vi "GCSArray_regex_string.vi"(0 "Selector":T1, 5 "error in (no error)":errorcluster) -> (14 "Regex string":string, 19 "error out":errorcluster)   [LabVIEW 2026]
doc: "Translates a GCSArray_regex_selector value into its corresponding regular expression string (regex). These text string expressions are used to filter, cut and select text areas in GCS arrays with the LabVIEW regular expression engine.\n\nFor details on how it works, please visit:\nhttps://zone.ni.com/reference/en-XX/help/371361L-01/glang/match_regular_expression/"
uses:
  GCSArray_regex_selector.ctl
panel:
  # "Translate a GCSArray selector enum value into the\ncorresponding regular expression string."
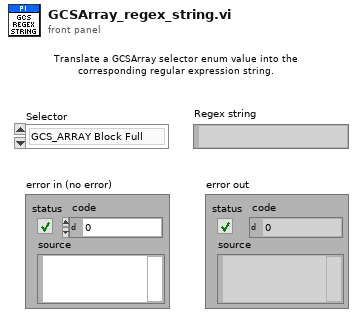
[diagram p1: front panel]
types:
  T1 = typedef "GCSArray_regex_selector.ctl" = enum16{"GCS_ARRAY Block Full", "GCS_ARRAY Block ID", "GCS_ARRAY Block Header", "GCS_ARRAY Block Data", "GCS_ARRAY Identifier", "GCS_ARRAY Remark", "GCS_ARRAY Version", "GCS_ARRAY Dimension", "GCS_ARRAY Type", "GCS_ARRAY Separator", "GCS_ARRAY NData", "GCS_ARRAY NData%", "GCS_ARRAY NData% Keyword", "GCS_ARRAY Name%", "GCS_ARRAY Name% Keyword", "GCS_ARRAY Start%", "GCS_ARRAY Start% Keyword", "GCS_ARRAY End%", "GCS_ARRAY End% Keyword", "GCS_ARRAY Delta%", "GCS_ARRAY Delta% Keword", "GCS_ARRAY Sample Time", "GCS_ARRAY Unit of transmitted value%", "GCS_ARRAY Trans_Unit% Keyword", "GCS_ARRAY Trans_Unit% = RAW Keyword", "GCS_ARRAY Unit of displayed value%", "GCS_ARRAY Disp_Unit% Keyword", "GCS_ARRAY Nominator%", "GCS_ARRAY Ratio_Nom% Keyword", "GCS_ARRAY Denominator%", "GCS_ARRAY Ratio_Denom% Keyword", "GCS_ARRAY End of Header", "GCS_ARRAY Empty line of Header"}
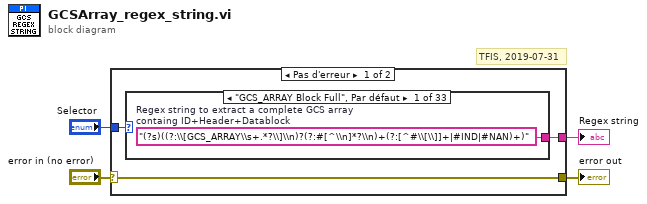
[diagram p0: block diagram]
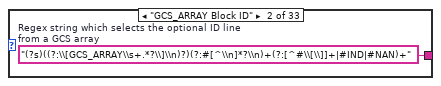
[diagram p2: hidden frame]
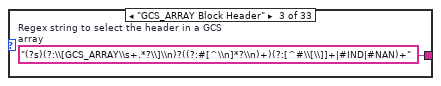
[diagram p3: hidden frame]
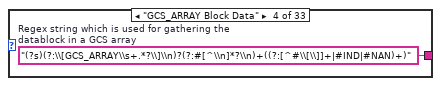
[diagram p4: hidden frame]
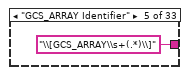
[diagram p5: hidden frame]
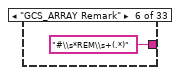
[diagram p6: hidden frame]
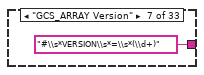
[diagram p7: hidden frame]
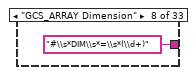
[diagram p8: hidden frame]
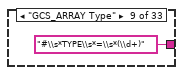
[diagram p9: hidden frame]
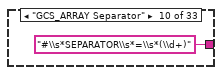
[diagram p10: hidden frame]
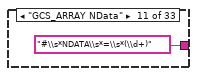
[diagram p11: hidden frame]
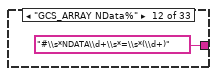
[diagram p12: hidden frame]
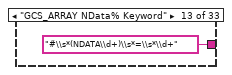
[diagram p13: hidden frame]
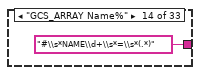
[diagram p14: hidden frame]
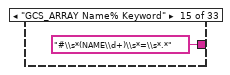
[diagram p15: hidden frame]
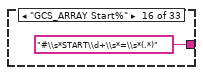
[diagram p16: hidden frame]
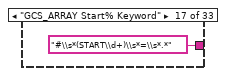
[diagram p17: hidden frame]
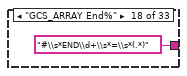
[diagram p18: hidden frame]
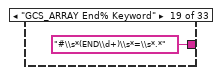
[diagram p19: hidden frame]
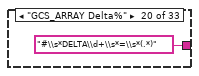
[diagram p20: hidden frame]
diagram:
  # "TFIS, 2019-07-31"
  n1 = case shown="Pas d'erreur" "error in (no error)" {
    selector: "error in (no error)" -> [w6 w42]
    tunnel: [w6 w42] -> w4
    tunnel: [w7 ""] -> w3
    tunnel: "Selector" -> [w5 _]
    frame No Error {
      n2 = case shown="\"GCS_ARRAY Block Full\", Par défaut" w5 {
        tunnel: [w8 w9 w10 w11 "\\[GCS_ARRAY\\s+(.*)\\]" "#\\s*REM\\s+(.*)" "#\\s*VERSION\\s*=\\s*(\\d+)" "#\\s*DIM\\s*=\\s*(\\d+)" "#\\s*TYPE\\s*=\\s*(\\d+)" "#\\s*SEPARATOR\\s*=\\s*(\\d+)" "#\\s*NDATA\\s*=\\s*(\\d+)" "#\\s*NDATA\\d+\\s*=\\s*(\\d+)" "#\\s*(NDATA\\d+)\\s*=\\s*\\d+" "#\\s*NAME\\d+\\s*=\\s*(.*)" "#\\s*(NAME\\d+)\\s*=\\s*.*" "#\\s*START\\d+\\s*=\\s*(.*)" "#\\s*(START\\d+)\\s*=\\s*.*" "#\\s*END\\d+\\s*=\\s*(.*)" "#\\s*(END\\d+)\\s*=\\s*.*" "#\\s*DELTA\\d+\\s*=\\s*(.*)" "#\\s*(DELTA\\d+)\\s*=\\s*.*" "#\\s*SAMPLE_TIME\\s*=\\s*(.*)" "#\\s*TRANS_UNIT\\d+\\s*=\\s*(.*)" "#\\s*(TRANS_UNIT\\d+)\\s*=\\s*.*" "#\\s*(TRANS_UNIT\\d+)\\s*=\\s*RAW" "#\\s*DISP_UNIT\\d+\\s*=\\s*(.*)" "#\\s*(DISP_UNIT\\d+)\\s*=\\s*.*" "#\\s*RATIO_NOM\\d+\\s*=\\s*(.*)" "#\\s*(RATIO_NOM\\d+)\\s*=\\s*.*" "#\\s*RATIO_DENOM\\d+\\s*=\\s*(.*)" "#\\s*(RATIO_DENOM\\d+)\\s*=\\s*.*" "(#\\s*END_HEADER)" "(#\\s*\\n+)"] -> w7
        frame "GCS_ARRAY Block Full", Default {
          w8 = "(?s)((?:\\[GCS_ARRAY\\s+.*?\\]\\n)?(?:#[^\\n]*?\\n)+(?:[^#\\[\\]]+|#IND|#NAN)+)"  # Regex string to extract a complete GCS array containg ID+Header+Datablock
        }
        frame "GCS_ARRAY Block ID" {
          w9 = "(?s)((?:\\[GCS_ARRAY\\s+.*?\\]\\n)?)(?:#[^\\n]*?\\n)+(?:[^#\\[\\]]+|#IND|#NAN)+"  # Regex string which selects the optional ID line from a GCS array
        }
        frame "GCS_ARRAY Block Header" {
          w10 = "(?s)(?:\\[GCS_ARRAY\\s+.*?\\]\\n)?((?:#[^\\n]*?\\n)+)(?:[^#\\[\\]]+|#IND|#NAN)+"  # Regex string to select the header in a GCS array
        }
        frame "GCS_ARRAY Block Data" {
          w11 = "(?s)(?:\\[GCS_ARRAY\\s+.*?\\]\\n)?(?:#[^\\n]*?\\n)+((?:[^#\\[\\]]+|#IND|#NAN)+)"  # Regex string which is used for gathering the datablock in a GCS array
        }
        frame "GCS_ARRAY Identifier" {
        }
        frame "GCS_ARRAY Remark" {
        }
        frame "GCS_ARRAY Version" {
        }
        frame "GCS_ARRAY Dimension" {
        }
        frame "GCS_ARRAY Type" {
        }
        frame "GCS_ARRAY Separator" {
        }
        frame "GCS_ARRAY NData" {
        }
        frame "GCS_ARRAY NData%" {
        }
        frame "GCS_ARRAY NData% Keyword" {
        }
        frame "GCS_ARRAY Name%" {
        }
        frame "GCS_ARRAY Name% Keyword" {
        }
        frame "GCS_ARRAY Start%" {
        }
        frame "GCS_ARRAY Start% Keyword" {
        }
        frame "GCS_ARRAY End%" {
        }
        frame "GCS_ARRAY End% Keyword" {
        }
        frame "GCS_ARRAY Delta%" {
        }
        frame "GCS_ARRAY Delta% Keword" {
        }
        frame "GCS_ARRAY Sample Time" {
        }
        frame "GCS_ARRAY Unit of transmitted value%" {
        }
        frame "GCS_ARRAY Trans_Unit% Keyword" {
        }
        frame "GCS_ARRAY Trans_Unit% = RAW Keyword" {
        }
        frame "GCS_ARRAY Unit of displayed value%" {
        }
        frame "GCS_ARRAY Disp_Unit% Keyword" {
        }
        frame "GCS_ARRAY Nominator%" {
        }
        frame "GCS_ARRAY Ratio_Nom% Keyword" {
        }
        frame "GCS_ARRAY Denominator%" {
        }
        frame "GCS_ARRAY Ratio_Denom% Keyword" {
        }
        frame "GCS_ARRAY End of Header" {
        }
        frame "GCS_ARRAY Empty line of Header" {
        }
      }
    }
    frame Error {
    }
  }
  "Regex string" <- w3
  "error out" <- w4
